vi "LSMcontroller_v57.vi"() -> ()   [LabVIEW 2015] (continued)
                                n403 = Boolean Array To Number(Boolean array=w2608) -> (number=w2607:u32)
                                n404 = case shown="2" w2607 {
                                tunnel: w2604 -> [_ w2650 _ w2657]
                                tunnel: [_ w2649 _ w2655] -> w2603
                                frame 1 {
                                n405 = call "2pparameters.vi"("command"="get") -> ("params out"=w2615:T12)  [unwired: 1 in]
                                n406 = Unbundle By Name(w2615) -> ("wavdet"=w2616:bool, "sAOxy"=w2618:i32, "refwfsize"=w2619:dbl, "srate Img"=w2617:sgl)
                                n407 = call "waveformsDObuffer.vi"("command"="get") -> ("DO wf out"=w2611:digitalwaveform[])  [unwired: 1 in]
                                n408 = case shown="False" w2616 {
                                tunnel: [w2624 w2634] -> w2613
                                tunnel: w2617 -> [w2629 w2645]
                                tunnel: w2618 -> [w2623 w2638]
                                tunnel: w2619 -> [_ w2642]
                                frame False {
                                w2627 = u16 0 items=["unsigned binary", "offset binary", "2's complement"] ("data format (offset binary)")
                                n409 = Initialize Array(sgl 1.0, w2623) -> (w2620:sgl[])
                                n410 = Reciprocal(x=w2629) -> (1/x=w2630:sgl)
                                n411 = Bundle By Name("Y"=w2620, "dt"=w2630) -> (w2625:waveform(sgl))  [unwired: 1 in]
                                n412 = call-poly <vilib>:"Analog to Digital.vi"("data format (offset binary)"=w2627, "compress digital (T)"=TRUE, "full-scale range (pk-pk)"=1.0, "resolution (16 bit)"=1, "analog waveform"=w2625) -> ("digital waveform"=w2624:digitalwaveform)  [unwired: 3 in, 3 out]
                                }
                                frame True {
                                w2637 = u16 0 items=["unsigned binary", "offset binary", "2's complement"] ("data format (offset binary)")
                                n413 = To Double Precision Float(number=w2638) -> (double precision float=w2643:dbl)
                                n414 = Initialize Array(sgl 1.0, w2638) -> (w2631:sgl[])
                                n415 = Divide(x=w2642, y=w2643) -> (x/y=w2640:dbl)
                                n416 = Round Toward +Infinity(x=w2640) -> (ceil(x): smallest int >= x=w2641:dbl)
                                n417 = for {
                                N: w2641 -> [_]
                                tunnel: w2631 -> [w2647]
                                tunnel: [w2647] -> w2644 mode=concatenating
                                }
                                n418 = Reciprocal(x=w2645) -> (1/x=w2646:sgl)
                                n419 = Bundle By Name("Y"=w2644, "dt"=w2646) -> (w2635:waveform(sgl))  [unwired: 1 in]
                                n420 = call-poly <vilib>:"Analog to Digital.vi"("data format (offset binary)"=w2637, "compress digital (T)"=TRUE, "full-scale range (pk-pk)"=1.0, "resolution (16 bit)"=1, "analog waveform"=w2635) -> ("digital waveform"=w2634:digitalwaveform)  [unwired: 3 in, 3 out]
                                }
                                }
                                n421 = Build Array (concatenate)(w2611, w2613) -> (w2609:digitalwaveform[])
                                n422 = call "waveformsDObuffer.vi"("DO wf in"=w2609, "command"="set") -> ()  [unwired: 1 out]
                                }
                                frame 2 {
                                n423 = call "waveformsDObuffer.vi"("command"="get") -> ("DO wf out"=w2652:digitalwaveform[])  [unwired: 1 in]
                                n424 = Delete From Array(array=w2652, length=1, index=w2650) -> (deleted portion=w2649:digitalwaveform[], array with subset deleted=w2648:digitalwaveform[])
                                n425 = call "waveformsDObuffer.vi"("DO wf in"=w2648, "command"="set") -> ()  [unwired: 1 out]
                                }
                                frame 3, Default {
                                }
                                frame 0 {
                                n426 = call "2pparameters.vi"("command"="get") -> ("params out"=w2659:T12)  [unwired: 1 in]
                                n427 = Unbundle By Name(w2659) -> ("autoshutter"=w2658:bool, "wavdet"=w2656:bool)
                                n428 = case shown="True" w2658 {
                                tunnel: w2657 -> [_ w2663]
                                tunnel: w2656 -> [_ w2662]
                                tunnel: [_ w2661] -> w2655
                                frame False {
                                }
                                frame True {
                                n429 = case shown="False" w2662 {
                                tunnel: w2663 -> [w2667 _]
                                tunnel: [w2665 _] -> w2661
                                frame False {
                                w2674 = u16 0 items=["unsigned binary", "offset binary", "2's complement"] ("data format (offset binary)")
                                n430 = call "2pparameters.vi"("command"="get") -> ("params out"=w2681:T12)  [unwired: 1 in]
                                n431 = Unbundle By Name(w2681) -> ("sAOxy"=w2683:i32, "srate Img"=w2682:sgl)
                                n432 = call "waveformsDObuffer.vi"("command"="get") -> ("DO wf out"=w2668:digitalwaveform[])  [unwired: 1 in]
                                n433 = Index Array(array=w2668, index=w2667) -> (element=w2666:digitalwaveform)
                                n434 = Build Array(w2666) -> (w2665:digitalwaveform[])
                                n435 = Initialize Array(sgl 1.0, w2683) -> (w2669:sgl[])
                                n436 = Reciprocal(x=w2682) -> (1/x=w2676:sgl)
                                n437 = Bundle By Name("Y"=w2669, "dt"=w2676) -> (w2672:waveform(sgl))  [unwired: 1 in]
                                n438 = call-poly <vilib>:"Analog to Digital.vi"("data format (offset binary)"=w2674, "compress digital (T)"=TRUE, "full-scale range (pk-pk)"=1.0, "resolution (16 bit)"=1, "analog waveform"=w2672) -> ("digital waveform"=w2679:digitalwaveform)  [unwired: 3 in, 3 out]
                                n439 = Replace Array Subset(array=w2668, new element=w2679, index=w2667) -> (w2664:digitalwaveform[])
                                n440 = call "waveformsDObuffer.vi"("DO wf in"=w2664, "command"="set") -> ()  [unwired: 1 out]
                                }
                                frame True {
                                }
                                }
                                }
                                }
                                }
                                }
                              }
                              frame #8 {
                                n441 = Build Array(w2687, w2686) -> (w2689:bool[])
                                n442 = Boolean Array To Number(Boolean array=w2689) -> (number=w2688:u32)
                                n443 = case shown="0" w2688 {
                                tunnel: w2685 -> [_ w2715 _ w2727]
                                tunnel: [_ w2714 _ w2725] -> w2684
                                frame 1 {
                                w2702 = 0.0 ("DOtab")
                                n444 = call "2pparameters.vi"("command"="get") -> ("params out"=w2700:T12)  [unwired: 1 in]
                                n445 = call "waveformparamsv2.vi"("command"="get") -> ("Params out"=w2710:T16)  [unwired: 4 in, 2 out]
                                n446 = Unbundle By Name(w2710) -> ("DO parameters"=w2708:T19)
                                n447 = Unbundle By Name(w2700) -> ("srate"=w2697:sgl, "sAOxy"=w2699:i32)
                                n448 = To Double Precision Float(number=w2697) -> (double precision float=w2695:dbl)
                                n449 = To Double Precision Float(number=w2697) -> (double precision float=w2696:dbl)
                                n450 = To Double Precision Float(number=w2699) -> (double precision float=w2691:dbl)
                                n451 = Divide(x=w2696, y=w2691) -> (x/y=w2698:dbl)
                                n452 = Index Array(array=w2708, index=0) -> (element=w2707:T20)
                                n453 = Divide(x=1.0 ("Digital DC (%)"), y=w2691) -> (x/y=w2693:dbl)
                                n454 = Multiply(x=100.0, y=w2693) -> (x*y=w2690:dbl)
                                n455 = Bundle By Name(cluster=w2707, "Digital DC (%)"=w2690, "Digital phase"=w2702, "Digital Freq (Hz)"=w2698, "Sampling frequency (Hz)"=w2695, "Digital time offset (s)"=w2702, "padding value"=0.0, "matlab wave file"=path "LT", "DOtab"=0.0) -> (w2705:T20)
                                n456 = Build Array(w2705) -> (w2704:T19)
                                n457 = call "waveformparamsv2.vi"("command"="add DO", "add DO"=w2704) -> ()  [unwired: 3 in, 3 out]
                                }
                                frame 2 {
                                n458 = call "waveformparamsv2.vi"("command"="get") -> ("Params out"=w2717:T16)  [unwired: 4 in, 2 out]
                                n459 = in-place {
                                in-place-border: w2715 -> [w2721]
                                in-place-border: [w2720] -> w2714
                                n460 = in-place-cluster #8(w2717) -> ("DO parameters"=w2723:T19)
                                n461 = Delete From Array(array=w2723, length=1, index=w2721) -> (deleted portion=w2720:T19, array with subset deleted=w2722:T19)
                                n462 = in-place-cluster #8("DO parameters"=w2722) -> (w2716:T16)
                                }
                                n463 = call "waveformparamsv2.vi"("command"="set", "Params in"=w2716) -> ()  [unwired: 3 in, 3 out]
                                }
                                frame 3, Default {
                                }
                                frame 0 {
                                n464 = local read "Measurement"() -> (w2729:T5)
                                n465 = To Unsigned Long Integer(number=w2729) -> (unsigned 32bit integer=w2728:u32)
                                n466 = case shown="5..7" w2728 {
                                tunnel: w2727 -> [_ w2731]
                                tunnel: [_ w2730] -> w2726
                                frame 0..4, Default {
                                }
                                frame 5..7 {
                                n467 = stacked-sequence {
                                tunnel: w2731 -> [w2733 w2742]
                                tunnel: [w2732 _] -> w2730
                                frame #0 {
                                n468 = call "waveformparamsv2.vi"("command"="get") -> ("Params out"=w2735:T16)  [unwired: 4 in, 2 out]
                                n469 = Unbundle By Name(w2735) -> ("DO parameters"=w2736:T19)
                                n470 = Index Array(array=w2736, index=w2733) -> (element=w2732:T20)
                                }
                                frame #1 {
                                w2750 = 0.0 ("padding value")
                                n471 = call "2pparameters.vi"("command"="get") -> ("params out"=w2748:T12)  [unwired: 1 in]
                                n472 = Unbundle By Name(w2748) -> ("srate"=w2746:sgl, "sAOxy"=w2747:i32)
                                n473 = To Double Precision Float(number=w2746) -> (double precision float=w2744:dbl)
                                n474 = To Double Precision Float(number=w2746) -> (double precision float=w2745:dbl)
                                n475 = To Double Precision Float(number=w2747) -> (double precision float=w2740:dbl)
                                n476 = Divide(x=1.0 ("Digital DC (%)"), y=w2740) -> (x/y=w2739:dbl)
                                n477 = Multiply(x=100.0, y=w2739) -> (x*y=w2738:dbl)
                                n478 = Divide(x=w2745, y=w2740) -> (x/y=w2743:dbl)
                                n479 = call "replace DO wf param.vi"("Digital Freq (Hz)"=w2743, "Digital DC (%)"=w2738, "Digital phase"=w2750, "Sampling frequency (Hz)"=w2744, "Digital time offset (s)"=w2750, "index of DO wave"=w2742, "padding value"=w2750, "matlab wave file"=path "LT" ("matlab wave number")) -> ()  [unwired: 3 in]
                                }
                                }
                                }
                                }
                                n480 = Build Array(w2726) -> (w2725:T19)
                                }
                                }
                              }
                              frame #9 {
                                n481 = Build Array(w2755, w2754) -> (w2757:bool[])
                                n482 = Boolean Array To Number(Boolean array=w2757) -> (number=w2756:u32)
                                n483 = case shown="2" w2756 {
                                tunnel: w2753 -> [_ w2809 _ w2813]
                                tunnel: [_ w2804 _ w2810] -> w2752
                                frame 1 {
                                n484 = call "2pparameters.vi"("command"="get") -> ("params out"=w2764:T12)  [unwired: 1 in]
                                n485 = Unbundle By Name(w2764) -> ("wavdet"=w2765:bool, "sAOxy"=w2767:i32, "refwfsize"=w2768:dbl, "srate Img"=w2766:sgl)
                                n486 = call "waveformsDObuffer.vi"("command"="get") -> ("DO wf out"=w2760:digitalwaveform[])  [unwired: 1 in]
                                n487 = case shown="True" w2765 {
                                tunnel: [w2772 w2785] -> w2762
                                tunnel: w2766 -> [w2781 w2800]
                                tunnel: w2767 -> [w2771 w2791]
                                tunnel: w2768 -> [_ w2797]
                                frame False {
                                w2775 = u16 0 items=["unsigned binary", "offset binary", "2's complement"] ("data format (offset binary)")
                                n488 = Initialize Array(sgl 0.0, w2771) -> (w2778:sgl[])
                                n489 = Replace Array Subset(array=w2778, new element=sgl 1.0, index=0) -> (w2776:sgl[])
                                n490 = Reciprocal(x=w2781) -> (1/x=w2782:sgl)
                                n491 = Bundle By Name("Y"=w2776, "dt"=w2782) -> (w2773:waveform(sgl))  [unwired: 1 in]
                                n492 = call-poly <vilib>:"Analog to Digital.vi"("data format (offset binary)"=w2775, "compress digital (T)"=TRUE, "full-scale range (pk-pk)"=1.0, "resolution (16 bit)"=1, "analog waveform"=w2773) -> ("digital waveform"=w2772:digitalwaveform)  [unwired: 3 in, 3 out]
                                }
                                frame True {
                                w2788 = u16 0 items=["unsigned binary", "offset binary", "2's complement"] ("data format (offset binary)")
                                n493 = To Double Precision Float(number=w2791) -> (double precision float=w2798:dbl)
                                n494 = Initialize Array(sgl 0.0, w2791) -> (w2793:sgl[])
                                n495 = Divide(x=w2797, y=w2798) -> (x/y=w2795:dbl)
                                n496 = Round Toward +Infinity(x=w2795) -> (ceil(x): smallest int >= x=w2796:dbl)
                                n497 = Replace Array Subset(array=w2793, new element=sgl 1.0, index=0) -> (w2790:sgl[])
                                n498 = for {
                                N: w2796 -> [_]
                                tunnel: w2790 -> [w2802]
                                tunnel: [w2802] -> w2799 mode=concatenating
                                }
                                n499 = Reciprocal(x=w2800) -> (1/x=w2801:sgl)
                                n500 = Bundle By Name("Y"=w2799, "dt"=w2801) -> (w2786:waveform(sgl))  [unwired: 1 in]
                                n501 = call-poly <vilib>:"Analog to Digital.vi"("data format (offset binary)"=w2788, "compress digital (T)"=TRUE, "full-scale range (pk-pk)"=1.0, "resolution (16 bit)"=1, "analog waveform"=w2786) -> ("digital waveform"=w2785:digitalwaveform)  [unwired: 3 in, 3 out]
                                }
                                }
                                n502 = Build Array (concatenate)(w2760, w2762) -> (w2758:digitalwaveform[])
                                n503 = call "waveformsDObuffer.vi"("DO wf in"=w2758, "command"="set") -> ()  [unwired: 1 out]
                                }
                                frame 2 {
                                n504 = call "waveformsDObuffer.vi"("command"="get") -> ("DO wf out"=w2806:digitalwaveform[])  [unwired: 1 in]
                                n505 = Delete From Array(array=w2806, length=1, index=w2809) -> (deleted portion=w2804:digitalwaveform[], array with subset deleted=w2803:digitalwaveform[])
                                n506 = call "waveformsDObuffer.vi"("DO wf in"=w2803, "command"="set") -> ()  [unwired: 1 out]
                                }
                                frame 3, Default {
                                }
                                frame 0 {
                                n507 = local read "Measurement"() -> (w2812:T5)
                                n508 = To Unsigned Long Integer(number=w2812) -> (unsigned 32bit integer=w2811:u32)
                                n509 = case shown="5..7" w2811 {
                                tunnel: w2813 -> [_ w2816]
                                tunnel: [_ w2815] -> w2810
                                frame 0..4, Default {
                                }
                                frame 5..7 {
                                n510 = call "2pparameters.vi"("command"="get") -> ("params out"=w2823:T12)  [unwired: 1 in]
                                n511 = Unbundle By Name(w2823) -> ("wavdet"=w2824:bool, "sAOxy"=w2826:i32, "refwfsize"=w2827:dbl, "srate Img"=w2825:sgl)
                                n512 = call "waveformsDObuffer.vi"("command"="get") -> ("DO wf out"=w2817:digitalwaveform[])  [unwired: 1 in]
                                n513 = Index Array(array=w2817, index=w2816) -> (element=w2818:digitalwaveform)
                                n514 = case shown="True" w2824 {
                                tunnel: [w2831 w2844] -> w2821
                                tunnel: w2825 -> [w2840 w2859]
                                tunnel: w2826 -> [w2830 w2850]
                                tunnel: w2827 -> [_ w2856]
                                frame False {
                                w2834 = u16 0 items=["unsigned binary", "offset binary", "2's complement"] ("data format (offset binary)")
                                n515 = Initialize Array(sgl 0.0, w2830) -> (w2837:sgl[])
                                n516 = Replace Array Subset(array=w2837, new element=sgl 1.0, index=0) -> (w2835:sgl[])
                                n517 = Reciprocal(x=w2840) -> (1/x=w2841:sgl)
                                n518 = Bundle By Name("Y"=w2835, "dt"=w2841) -> (w2832:waveform(sgl))  [unwired: 1 in]
                                n519 = call-poly <vilib>:"Analog to Digital.vi"("data format (offset binary)"=w2834, "compress digital (T)"=TRUE, "full-scale range (pk-pk)"=1.0, "resolution (16 bit)"=1, "analog waveform"=w2832) -> ("digital waveform"=w2831:digitalwaveform)  [unwired: 3 in, 3 out]
                                }
                                frame True {
                                w2847 = u16 0 items=["unsigned binary", "offset binary", "2's complement"] ("data format (offset binary)")
                                n520 = To Double Precision Float(number=w2850) -> (double precision float=w2857:dbl)
                                n521 = Initialize Array(sgl 0.0, w2850) -> (w2852:sgl[])
                                n522 = Divide(x=w2856, y=w2857) -> (x/y=w2854:dbl)
                                n523 = Round Toward +Infinity(x=w2854) -> (ceil(x): smallest int >= x=w2855:dbl)
                                n524 = Replace Array Subset(array=w2852, new element=sgl 1.0, index=0) -> (w2849:sgl[])
                                n525 = for {
                                N: w2855 -> [_]
                                tunnel: w2849 -> [w2861]
                                tunnel: [w2861] -> w2858 mode=concatenating
                                }
                                n526 = Reciprocal(x=w2859) -> (1/x=w2860:sgl)
                                n527 = Bundle By Name("Y"=w2858, "dt"=w2860) -> (w2845:waveform(sgl))  [unwired: 1 in]
                                n528 = call-poly <vilib>:"Analog to Digital.vi"("data format (offset binary)"=w2847, "compress digital (T)"=TRUE, "full-scale range (pk-pk)"=1.0, "resolution (16 bit)"=1, "analog waveform"=w2845) -> ("digital waveform"=w2844:digitalwaveform)  [unwired: 3 in, 3 out]
                                }
                                }
                                n529 = Build Array(w2818) -> (w2815:digitalwaveform[])
                                n530 = Replace Array Subset(array=w2817, new element=w2821, index=w2816) -> (w2814:digitalwaveform[])
                                n531 = call "waveformsDObuffer.vi"("DO wf in"=w2814, "command"="set") -> ()  [unwired: 1 out]
                                }
                                }
                                }
                                }
                              }
                              frame #10 {
                                n532 = local read "Meastab"() -> (w2876:enum32{"X-Y Image", "Linescan", "Timetrace"})
                                n533 = property on="refwf" class="Ring (strict)"() -> ("RingText.Text"=w2873:string)  [unwired: 2 in, 2 out]
                                n534 = case shown="\"Timetrace\"" w2876 {
                                tunnel: [w2878 w2879] -> w2877
                                frame "X-Y Image", Default {
                                n535 = local read "Sampling rate"() -> (w2878:dbl)
                                }
                                frame "Timetrace" {
                                n536 = local read "srateAODOtt"() -> (w2879:dbl)
                                }
                                }
                                n537 = call "waveformsAObuffer.vi"("command"="get") -> ("AO wf out"=w2864:waveform(dbl)[])  [unwired: 1 in]
                                n538 = local read "wavdet"() -> (w2874:bool)
                                n539 = call "waveformsDObuffer.vi"("command"="get") -> ("DO wf out"=w2868:digitalwaveform[])  [unwired: 1 in]
                                n540 = call "correctwaveformsizetemp.vi"("new sampling frequency (Hz)"=w2877, "start"=TRUE, "reference waveforms to"=w2873, "Analog waveforms in"=w2864, "stop"=FALSE, "Digital waveforms in"=w2868) -> ("analog wf out"=w2870:waveform(dbl)[], "Digital wf out"=w2872:digitalwaveform[], "measpoints"=w2875:i32)
                                n541 = call "GetNumCamFramesv2.vi"("Digital Waveform Graph"=w2872) -> ("Numeric"=w2871:i32)  [unwired: 10 in]
                                n542 = call "waveformsDObuffer.vi"("DO wf in"=w2872, "command"="set") -> ()  [unwired: 1 out]
                                n543 = call "waveformsAObuffer.vi"("AO wf in"=w2870, "command"="set") -> ()  [unwired: 1 out]
                                n544 = local write "Total Camera Frames"(w2871) -> ()
                                n545 = case shown="True" w2874 {
                                tunnel: w2875 -> [_ w2880]
                                frame False {
                                }
                                frame True {
                                n546 = local write "# of frames"(w2880) -> ()
                                }
                                }
                              }
                            }
                          }
                          frame #6 {
                            # "Disabled for conversion to 64 bit"
                            n547 = disable-structure shown="Disabled" {
                              frame Disabled {
                                n548 = local read "Measurement"() -> (w2885:T5)
                                n549 = case shown="\"Lifetime (scan)\"" w2885 {
                                frame "X-Y-t movie", Default {
                                }
                                frame "Lifetime (scan)" {
                                # "total acquisition time"
                                n550 = call "2pparameters.vi"("command"="get") -> ("params out"=w2891:T12)  [unwired: 1 in]
                                n551 = Unbundle By Name(w2891) -> ("measpoints"=w2912:i32, "avpp"=w2913:i32, "sAOxy"=w2892:i32, "srate Img"=w2914:sgl)
                                n552 = Multiply(x=w2912, y=w2913) -> (x*y=w2910:i32)
                                n553 = To Double Precision Float(number=w2892) -> (double precision float=w2897:dbl)
                                n554 = Divide(x=w2897, y=w2914) -> (x/y=w2899:dbl)
                                n555 = To Double Precision Float(number=w2910) -> (double precision float=w2895:dbl)
                                n556 = local read "min phot"() -> (w2906:u32)
                                n557 = local read "expected c/s"() -> (w2907:dbl)
                                n558 = Multiply(x=w2895, y=w2899) -> (x*y=w2893:dbl)
                                n559 = Multiply(x=w2893, y=1000.0) -> (x*y=w2898:dbl)
                                n560 = local read "Ch1 ZeroX"() -> (w2904:i32)
                                n561 = local read "truncate"() -> (w2905:u32)
                                n562 = To Long Integer(number=w2898) -> (32bit integer=w2908:i32)
                                n563 = To Long Integer(number=w2907) -> (32bit integer=w2909:i32)
                                n564 = local read "Number of Bins"() -> (w2900:u32)
                                n565 = local read "Ch1 Level"() -> (w2902:i32)
                                n566 = local read "Ch0 ZeroX"() -> (w2903:i32)
                                n567 = local write "Acquisition time"(w2908) -> ()
                                n568 = local read "Ch0 Level"() -> (w2901:i32)
                                n569 = call "lifetimeparameters.vi"("command"="get") -> ("Params out"=w2889:T21)  [unwired: 1 in]
                                n570 = Add(x=10, y=w2908) -> (x+y=w2896:i32)
                                n571 = Bundle By Name(cluster=w2889, "acq time"=w2896, "acq rate"=w2909, "# bins"=w2900, "Ch0 Level"=w2901, "Ch1 Level"=w2902, "Ch0 ZeroX"=w2903, "Ch1 ZeroX"=w2904, "min photons"=w2906, "truncate"=w2905) -> (w2888:T21)
                                n572 = local write "Acquisition rate"(w2909) -> ()
                                n573 = call "lifetimeparameters.vi"("Params in"=w2888, "command"="set") -> ()  [unwired: 1 out]
                                }
                                }
                                n574 = local read "min phot"() -> (w2883:u32)
                                n575 = Decrement(x=w2883) -> (x-1=w2884:u32)
                                n576 = To Double Precision Float(number=w2884) -> (double precision float=w2882:dbl)
                                n577 = property on="img_CH1" class="IntGraph (strict)"("ZScale.Minimum"=w2882) -> ()  [unwired: 2 in, 2 out]
                              }
                              frame Enabled {
                              }
                            }
                            n578 = local write "64bit disabled"(TRUE ("64bit disabled")) -> ()
                          }
                          frame #7 {
                            n579 = local read "Sampling rate"() -> (w2916:dbl)
                            n580 = call "calcdaqtime.vi"("sampling rate"=w2916) -> ("Calc. time per frame (ms)"=w2915:dbl)
                            n581 = local write "Calc. time per frame (ms)"(w2915) -> ()
                          }
                          frame #8 {
                            n582 = call "2pparameters.vi"("command"="get") -> ("params out"=w2927:T12)  [unwired: 1 in]
                            n583 = local read "Measurement"() -> (w2918:T5)
                            n584 = Unbundle By Name(w2927) -> ("bufferAI"=w2925:i32, "srate"=w2926:sgl)
                            n585 = To Double Precision Float(number=w2925) -> (double precision float=w2919:dbl)
                            n586 = To Double Precision Float(number=w2926) -> (double precision float=w2929:dbl)
                            n587 = case shown="\"X-Y-t movie\", Default" w2918 {
                              tunnel: [w2934 w2938] -> w2917
                              frame "X-Y-t movie", Default {
                                n588 = local read "wavdet"() -> (w2935:bool)
                                n589 = case shown="False" w2935 {
                                tunnel: [w2936 w2937] -> w2934
                                frame False {
                                w2936 = 10123 items=["Finite Samples"=10178, "Continuous Samples"=10123, "Hardware Timed Single Point"=12522] ("sample mode")
                                }
                                frame True {
                                w2937 = 10123 items=["Finite Samples"=10178, "Continuous Samples"=10123, "Hardware Timed Single Point"=12522] ("sample mode")
                                }
                                }
                              }
                              frame "X-Y-Z stack" {
                                w2938 = 10178 items=["Finite Samples"=10178, "Continuous Samples"=10123, "Hardware Timed Single Point"=12522] ("sample mode")
                              }
                            }
                            n590 = Divide(x=w2919, y=w2929) -> (x/y=w2933:dbl)
                            n591 = Multiply(x=w2933, y=2.0) -> (x*y=w2930:dbl)
                            n592 = Max & Min(x=w2930, y=10.0) -> (max(x,y)=w2920:dbl)  [unwired: 1 out]
                            n593 = call "2pparameters.vi"("command"="get") -> ("params out"=w2924:T12)  [unwired: 1 in]
                            n594 = Bundle By Name(cluster=w2924, "timeout"=w2920, "sample mode"=w2917) -> (w2921:T12)
                            n595 = call "2pparameters.vi"("Params in"=w2921, "command"="set") -> ()  [unwired: 1 out]
                          }
                          frame #9 {
                            n596 = local read "# of frames"() -> (w2939:i32)
                            n597 = call "timestamps.vi"("# of frames"=w2939, "command"="init") -> ()  [unwired: 2 in, 1 out]
                          }
                        }
                      }
                      frame #2 {
                        # "Disabled for conversion to 64 bit"
                        n598 = call "prepAO_img.vi"() -> ("Terminal Name with Device Prefix"=w2942:tag)
                        n599 = call "prepAI_img.vi"("triggersource"=w2942) -> ()  [unwired: 2 in]
                        n600 = call "prepCI_img.vi"("ArmStart.DigEdge.Src"=w2942) -> ()  [unwired: 1 in]
                        n601 = call "prepDO_img.vi"() -> ()  [unwired: 2 in]
                        n602 = disable-structure shown="Disabled" {
                          frame Disabled {
                            n603 = local read "Measurement"() -> (w2943:T5)
                            n604 = case shown="\"Lifetime (scan)\"" w2943 {
                              frame "X-Y-t movie", Default {
                              }
                              frame "Lifetime (scan)" {
                                n605 = stacked-sequence {
                                frame #0 {
                                n606 = call "PH-temp.vi"("String"="clear" ("command")) -> ()  [unwired: 2 in, 2 out]
                                n607 = call "PH-temp-raw.vi"("command"="empty") -> ()  [unwired: 1 in, 1 out]
                                }
                                frame #1 {
                                n608 = call "calib.vi"() -> ()  [unwired: 1 in]
                                }
                                frame #2 {
                                n609 = call "setup.vi"() -> ()  [unwired: 1 in]
                                }
                                }
                              }
                            }
                          }
                          frame Enabled {
                          }
                        }
                        n610 = local write "64bit disabled"(TRUE ("64bit disabled")) -> ()
                      }
                      frame #3 {
                        n611 = local read "save\ndata"() -> (w2946:bool)
                        n612 = case shown="True" w2946 {
                          tunnel: w2947 -> [_ w2951]
                          frame False {
                          }
                          frame True {
                            n613 = local read "filename prefix"() -> (w2949:string)
                            n614 = local read "data dir"() -> (w2950:path)
                            n615 = call "preparetiffs.vi"("filename prefix"=w2949, "data dir"=w2950, "timestamp"=w2951) -> ("full-filename"=w2948:string)  [unwired: 1 in]
                            n616 = local write "full-filename"(w2948) -> ()
                          }
                        }
                        n617 = call "preptempbuffers.vi"() -> ()  [unwired: 12 in]
                      }
                      frame #4 {
                        # "Disabled Thorlabs Zstage;\nneeds to be replaced by PI code"
                        n618 = disable-structure shown="Disabled" {
                          frame Disabled {
                            n619 = local read "Measurement"() -> (w2953:T5)
                            n620 = case shown="\"X-Y-Z stack\"" w2953 {
                              frame "X-Y-t movie", Default {
                              }
                              frame "X-Y-Z stack" {
                                n621 = local read "Z-Start (um)"() -> (w2964:dbl)
                                n622 = local read "Z-end (um)"() -> (w2963:dbl)
                                n623 = local read "# of frames"() -> (w2965:i32)
                                n624 = call "2pparameters.vi"("command"="get") -> ("params out"=w2956:T12)  [unwired: 1 in]
                                n625 = Unbundle By Name(w2956) -> ("motorref"=w2955:refnum<k7>)
                                n626 = call "calcZslice.vi"("current slice"=0, "# of Slices"=w2965, "Z-Start (um)"=w2964, "Z-end (um)"=w2963) -> ("zpos (mm)"=w2958:sgl)
                                n627 = call "MoveZ.vi"("RetPos"=TRUE, "Wait"=TRUE, "GoTo (mm)"=w2958, "MG17Motor"=w2955) -> ("EndPosition (um)"=w2962:sgl)  [unwired: 1 out]
                                n628 = Multiply(x=w2958, y=sgl 1000.0) -> (x*y=w2959:sgl)
                                n629 = local write "Actual Z position"(w2962) -> ()
                                n630 = local write "Cal. Z"(w2959) -> ()
                              }
                            }
                          }
                          frame Enabled {
                          }
                        }
                        n631 = local write "Thorlabs Zstage disabled"(TRUE ("64bit disabled")) -> ()
                      }
                      frame #5 {
                        n632 = flat-sequence {
                          frame #0 {
                            n633 = call "2pparameters.vi"("command"="get") -> ("params out"=w2968:T12)  [unwired: 1 in]
                            n634 = Unbundle By Name(w2968) -> ("autoshutter"=w2969:bool)
                            n635 = case shown="True" w2969 {
                              frame False {
                              }
                              frame True {
                                n636 = call "shuttercontrol.vi"("command"="open") -> ()  [unwired: 1 in, 1 out]
                              }
                            }
                          }
                          frame #1 {
                            n637 = call "2pparameters.vi"("command"="get") -> ("params out"=w2973:T12)  [unwired: 1 in]
                            n638 = Tick Count (ms)() -> (millisecond timer value=w2972:u32)
                            n639 = Bundle By Name(cluster=w2973, "starttick"=w2972) -> (w2971:T12)
                            n640 = call "2pparameters.vi"("Params in"=w2971, "command"="set") -> ()  [unwired: 1 out]
                          }
                        }
                      }
                      frame #6 {
                        n641 = local read "Measurement"() -> (w2976:T5)
                        n642 = case shown="\"Lifetime (scan)\"" w2976 {
                          frame "X-Y-t movie" {
                            n643 = flat-sequence {
                              frame #0 {
                                n644 = call "runAI_img.vi"() -> ()  [unwired: 12 in]
                                n645 = call "runCI.vi"() -> ()  [unwired: 12 in]
                                n646 = call "runDO_img.vi"() -> ()  [unwired: 12 in]
                              }
                              frame #1 {
                                n647 = call "runAO_img.vi"() -> ()  [unwired: 12 in]
                              }
                            }
                          }
                          frame "Lifetime (scan)" {
                            # "Disabled for conversion to 64 bit"
                            n648 = disable-structure shown="Disabled" {
                              frame Disabled {
                                n649 = flat-sequence {
                                frame #0 {
                                n650 = call "runLT_img.vi"() -> ()  [unwired: 1 in]
                                n651 = call "runDO_img.vi"() -> ()  [unwired: 12 in]
                                }
                                frame #1 {
                                n652 = call "runAI_img.vi"() -> ()  [unwired: 12 in]
                                n653 = call "runCI.vi"() -> ()  [unwired: 12 in]
                                }
                                frame #2 {
                                n654 = call "runAO_img.vi"() -> ()  [unwired: 12 in]
                                }
                                }
                              }
                              frame Enabled {
                              }
                            }
                            n655 = local write "64bit disabled"(TRUE ("64bit disabled")) -> ()
                          }
                          frame "X-Y-Z stack", Default {
                          }
                        }
                      }
                      frame #7 {
                        # "Disabled for conversion to 64 bit"
                        n656 = while {
                          i -> [w3005]
                          stop <- w3002 stop-if-true
                          n657 = local read "Exit"() -> (w3010:bool)
                          n658 = local read "Stop"() -> (w3001:bool)
                          n659 = Or(x=w3001, y=w3010) -> (x .or. y?=w3006:bool)
                          n660 = case shown="False" w3006 {
                            tunnel: w3005 -> [w3011 _]
                            frame False {
                              n661 = stacked-sequence {
                                seq-local: [w3013 _ _ _ _ _ _] -> [_ _ _ _ _ _ w3138]
                                seq-local: [w3012 _ _ _ _ _ _] -> [_ _ _ _ _ _ w3137]
                                tunnel: w3011 -> [_ w3018 _ _ _ _ _]
                                frame #0 {
                                n662 = local read "Live"() -> (w3014:bool)
                                n663 = case shown="True" w3014 {
                                tunnel: [_ w3016] -> w3013
                                tunnel: [_ w3015] -> w3012
                                frame False {
                                }
                                frame True {
                                n664 = local read "Laserpower \n(%)"() -> (w3015:dbl)
                                n665 = local read "lpow"() -> (w3016:dbl)
                                }
                                }
                                n666 = call "preptempbuffers.vi"() -> ()  [unwired: 12 in]
                                }
                                frame #1 {
                                # "Disabled Thorlabs Zstage;\nneeds to be replaced by PI code"
                                n667 = disable-structure shown="Disabled" {
                                disable-tunnel: w3018 -> [w3019 _]
                                frame Disabled {
                                # "Move in Z if necessary"
                                n668 = local read "Measurement"() -> (w3020:T5)
                                n669 = case shown="\"X-Y-Z stack\"" w3020 {
                                tunnel: w3019 -> [_ w3024]
                                frame "X-Y-t movie", Default {
                                }
                                frame "X-Y-Z stack" {
                                n670 = local read "Z-Start (um)"() -> (w3031:dbl)
                                n671 = local read "Z-end (um)"() -> (w3030:dbl)
                                n672 = local read "# of frames"() -> (w3032:i32)
                                n673 = call "2pparameters.vi"("command"="get") -> ("params out"=w3022:T12)  [unwired: 1 in]
                                n674 = Unbundle By Name(w3022) -> ("motorref"=w3021:refnum<k7>)
                                n675 = call "calcZslice.vi"("current slice"=w3024, "# of Slices"=w3032, "Z-Start (um)"=w3031, "Z-end (um)"=w3030) -> ("zpos (mm)"=w3025:sgl)
                                n676 = call "MoveZ.vi"("RetPos"=TRUE, "Wait"=TRUE, "GoTo (mm)"=w3025, "MG17Motor"=w3021) -> ("EndPosition (um)"=w3029:sgl)  [unwired: 1 out]
                                n677 = Multiply(x=w3025, y=sgl 1000.0) -> (x*y=w3026:sgl)
                                n678 = local write "Actual Z position"(w3029) -> ()
                                n679 = local write "Cal. Z"(w3026) -> ()
                                }
                                }
                                }
                                frame Enabled {
                                }
                                }
                                n680 = local write "Thorlabs Zstage disabled"(TRUE ("64bit disabled")) -> ()
                                }
                                frame #2 {
                                # "main loop"
                                n681 = for {
                                N: "avpp" -> [_]
                                i -> [w3039]
                                n682 = local read "Stop"() -> (w3037:bool)
                                n683 = local read "Exit"() -> (w3036:bool)
                                n684 = Increment(x=w3039) -> (x+1=w3038:i32)
                                n685 = Or(x=w3037, y=w3036) -> (x .or. y?=w3035:bool)
                                n686 = case shown="False" w3035 {
                                tunnel: w3038 -> [w3040 _]
                                frame False {
                                n687 = stacked-sequence {
                                seq-local: [w3041 _ _ _ _ _ _] -> [_ _ _ w3054 w3066 w3074 _]
                                tunnel: w3040 -> [w3042 _ _ _ _ _ _]
                                frame #0 {
                                n688 = local read "Live"() -> (w3041:bool)
                                n689 = case shown="True" w3041 {
                                tunnel: w3042 -> [_ w3045]
                                frame False {
                                }
                                frame True {
                                # "collect timetag for current image\nplus curent average"
                                n690 = To Single Precision Float(number=w3045) -> (single precision float=w3043:sgl)
                                n691 = Tick Count (ms)() -> (millisecond timer value=w3044:u32)
                                n692 = local write "Tick for Frame"(w3044) -> ()
                                n693 = local write "Current Average"(w3043) -> ()
                                }
                                }
                                }
                                frame #1 {
                                n694 = local read "Measurement"() -> (w3046:T5)
                                n695 = case shown="\"X-Y-Z stack\"" w3046 {
                                frame "X-Y-t movie", Default {
                                }
                                frame "X-Y-Z stack" {
                                n696 = stacked-sequence {
                                frame #0 {
                                n697 = disable-structure shown="Disabled" {
                                frame Disabled {
                                n698 = call "2pparameters.vi"("command"="get") -> ("params out"=w3048:T12)  [unwired: 1 in]
                                n699 = Unbundle By Name(w3048) -> ("autoshutter"=w3049:bool)
                                n700 = case shown="True" w3049 {
                                frame False {
                                }
                                frame True {
                                n701 = call "shuttercontrol.vi"("command"="open") -> ()  [unwired: 1 in, 1 out]
                                }
                                }
                                }
                                frame Enabled {
                                }
                                }
                                }
                                frame #1 {
                                n702 = call "runAI_img.vi"() -> ()  [unwired: 12 in]
                                n703 = call "runCI.vi"() -> ()  [unwired: 12 in]
                                n704 = call "runDO_img.vi"() -> ()  [unwired: 12 in]
                                }
                                frame #2 {
                                n705 = call "runAO_img.vi"() -> ()  [unwired: 12 in]
                                }
                                }
                                }
                                }
                                }
                                frame #2 {
                                n706 = call "collectCI_img.vi"() -> ("Avg cts/s"=w3053:dbl, "recorded samples"=w3052:i32)  [unwired: 1 out]
                                n707 = call "collectAI_img.vi"() -> ("wrap"=w3051:i32)  [unwired: 3 in]
                                n708 = local write "scol"(w3052) -> ()
                                n709 = local write "wrap"(w3051) -> ()
                                n710 = local write "Avg Counts/s"(w3053) -> ()
                                }
                                frame #3 {
                                n711 = case shown="True" w3054 {
                                frame False {
                                }
                                frame True {
                                n712 = local read "Measurement"() -> (w3055:T5)
                                n713 = case shown="\"X-Y-t movie\", Default" w3055 {
                                frame "X-Y-t movie", Default {
                                n714 = local read "ROI Type"() -> (w3056:u16)
                                n715 = case shown="0" w3056 {
                                frame 0 {
                                # "display chosen channels"
                                n716 = local read "Current Average"() -> (w3065:sgl)
                                n717 = local read "image1list"() -> (w3061:u16)
                                n718 = local read "image2list"() -> (w3064:u16)
                                n719 = To Unsigned Word Integer(number=w3064) -> (unsigned 16bit integer=w3059:u16)
                                n720 = To Unsigned Word Integer(number=w3061) -> (unsigned 16bit integer=w3060:u16)
                                n721 = call "dattoimage.vi"("image2list"=w3059, "Current Average"=w3065, "image1list"=w3060) -> ("image 2 array out"=w3063:sgl[][], "image 1 array out"=w3062:sgl[][])
                                n722 = Transpose 2D Array(2D array=w3062) -> (transposed array=w3058:sgl[][])
                                n723 = Transpose 2D Array(2D array=w3063) -> (transposed array=w3057:sgl[][])
                                n724 = local write "img_CH1"(w3058) -> ()
                                n725 = local write "img_CH2"(w3057) -> ()
                                }
                                frame 1, Default {
                                }
                                }
                                }
                                frame "Lifetime (scan)" {
                                }
                                }
                                }
                                }
                                }
                                frame #4 {
                                n726 = case shown="True" w3066 {
                                frame False {
                                }
                                frame True {
                                # "set colormaps"
                                n727 = call "misc-global.vi"("command"="get") -> ("misc out"=w3070:cluster{"Colormaps":u32[][]})  [unwired: 1 in]
                                n728 = Unbundle By Name(w3070) -> ("Colormaps"=w3069:u32[][])
                                n729 = control-ref of="img_CH1"() -> (w3073:refnum<vi>)
                                n730 = control-ref of="img_CH2"() -> (w3072:refnum<vi>)
                                n731 = Index Array(array=w3069, index (row)="Colormap") -> (element=w3068:u32[])  [unwired: 1 in]
                                n732 = property class="IntGraph (strict)"(reference=w3073, "Color Table"=w3068) -> ()  [unwired: 1 in, 2 out]
                                n733 = property class="IntGraph (strict)"(reference=w3072, "Color Table"=w3068) -> ()  [unwired: 1 in, 2 out]
                                }
                                }
                                }
                                frame #5 {
                                n734 = case shown="True" w3074 {
                                frame False {
                                }
                                frame True {
                                # "crude estimate of time per frame\n(resolution is 1 ms), not so much for\nplotting purposes, more for debugging\ncollection and processing data"
                                n735 = local read "ypixels ref"() -> (w3079:i32)
                                n736 = local read "Tick for Frame"() -> (w3080:u32)
                                n737 = Tick Count (ms)() -> (millisecond timer value=w3081:u32)
                                n738 = To Double Precision Float(number=w3079) -> (double precision float=w3078:dbl)
                                n739 = Subtract(x=w3081, y=w3080) -> (x-y=w3076:u32)
                                n740 = To Double Precision Float(number=w3076) -> (double precision float=w3077:dbl)
                                n741 = local write "Meas. time per frame (ms)"(w3076) -> ()
                                n742 = Divide(x=w3077, y=w3078) -> (x/y=w3075:dbl)
                                n743 = local write "time per line (ms)"(w3075) -> ()
                                }
                                }
                                }
                                frame #6 {
                                n744 = local read "Measurement"() -> (w3082:T5)
                                n745 = case shown="\"X-Y-Z stack\"" w3082 {
                                frame "X-Y-t movie", Default {
                                }
                                frame "X-Y-Z stack" {
                                n746 = call "2pparameters.vi"("command"="get") -> ("params out"=w3084:T12)  [unwired: 1 in]
                                n747 = Unbundle By Name(w3084) -> ("autoshutter"=w3085:bool)
                                n748 = call "stopCI_img.vi"() -> ()  [unwired: 12 in]
                                n749 = call "stopAI_img.vi"() -> ()  [unwired: 12 in]
                                n750 = case shown="True" w3085 {
                                frame False {
                                }
                                frame True {
                                n751 = call "shuttercontrol.vi"("command"="close") -> ()  [unwired: 1 in, 1 out]
                                }
                                }
                                n752 = Wait (ms)(milliseconds to wait=u32 100) -> ()  [unwired: 1 out]
                                n753 = call "stopAO_img.vi"() -> ()  [unwired: 12 in]
                                n754 = call "stopDO_img.vi"() -> ()  [unwired: 12 in]
                                }
                                }
                                }
                                }
                                }
                                frame True {
                                }
                                }
                                }
                                }
                                frame #3 {
                                n755 = local read "Measurement"() -> (w3088:T5)
                                n756 = case shown="\"Lifetime (scan)\"" w3088 {
                                frame "X-Y-t movie", Default {
                                }
                                frame "Lifetime (scan)" {
                                w3091 = u16 2 items=["Stream to disk", "Post process", "real time process"] ("Ring")
                                n757 = local read "T3R Data processing"() -> (w3092:u16)
                                n758 = Equal?(x=w3092, y=w3091) -> (x = y?=w3090:bool)
                                n759 = case shown="True" w3090 {
                                frame False {
                                }
                                frame True {
                                n760 = disable-structure shown="Disabled" {
                                frame Disabled {
                                n761 = local read "lineshift"() -> (w3095:i32)
                                n762 = call "wrapcutlifetime.vi"("lineshift"=w3095) -> ("pt3img"=w3097:u16[][], "lifetimes"=w3096:sgl[][], "okay"=w3093:bool, "# of frames"=w3094:i32)
                                n763 = case shown="True" w3093 {
                                tunnel: w3097 -> [_ w3107]
                                tunnel: w3096 -> [_ w3105]
                                tunnel: w3094 -> [_ w3101]
                                frame False {
                                }
                                frame True {
                                # "lifetime"
                                # "intensity"
                                n764 = Transpose 2D Array(2D array=w3107) -> (transposed array=w3099:u16[][])
                                n765 = Transpose 2D Array(2D array=w3105) -> (transposed array=w3106:sgl[][])
                                n766 = local write "frames recorded"(w3101) -> ()
                                n767 = local read "counts"() -> (w3100:i32)
                                n768 = Array Max & Min(array=w3099) -> (max value=w3104:u16)  [unwired: 3 out]
                                n769 = To Single Precision Float(number=w3099) -> (single precision float=w3098:sgl[][])
                                n770 = local write "img_CH2"(w3106) -> ()
                                n771 = local write "img_CH1"(w3098) -> ()
                                n772 = Quotient & Remainder(x=w3100, y=w3101) -> (floor(x/y)=→"photons/frame":i32)  [unwired: 1 out]
                                n773 = To Double Precision Float(number=w3104) -> (double precision float=w3103:dbl)
                                n774 = property on="img_CH1" class="IntGraph (strict)"("ZScale.Maximum"=w3103) -> ()  [unwired: 2 in, 2 out]
                                }
                                }
                                }
                                frame Enabled {
                                }
                                }
                                }
                                }
                                }
                                }
                                n775 = local read "save\ndata"() -> (w3089:bool)
                                n776 = case shown="True" w3089 {
                                frame False {
                                }
                                frame True {
                                n777 = local read "Current Average"() -> (w3108:sgl)
                                n778 = call "savetiffs.vi"("current average"=w3108) -> ()
                                }
                                }
                                }
                                frame #4 {
                                n779 = local read "save\ndata"() -> (w3109:bool)
                                n780 = case shown="True" w3109 {
                                frame False {
                                }
                                frame True {
                                n781 = local read "points recorded"() -> (w3111:i32)
                                n782 = call "timestamps.vi"("points recorded"=w3111, "command"="add") -> ()  [unwired: 2 in, 1 out]
                                }
                                }
                                }
                                frame #5 {
                                n783 = local read "Live"() -> (w3112:bool)
                                n784 = case shown="True" w3112 {
                                frame False {
                                }
                                frame True {
                                n785 = local read "downright"() -> (w3117:bool)
                                n786 = local read "downleft"() -> (w3119:bool)
                                n787 = local read "upright"() -> (w3115:bool)
                                n788 = local read "upleft"() -> (w3113:bool)
                                n789 = local read "down"() -> (w3118:bool)
                                n790 = local read "right"() -> (w3116:bool)
                                n791 = local read "left"() -> (w3120:bool)
                                n792 = local read "up"() -> (w3114:bool)
                                n793 = Compound Arithmetic op=OR(w3113, w3114, w3115, w3116, w3117, w3118, w3119, w3120) -> (w3121:bool)
                                n794 = case shown="True" w3121 {
                                frame False {
                                }
                                frame True {
                                n795 = stacked-sequence {
                                frame #0 {
                                n796 = local read "downright"() -> (w3123:bool)
                                n797 = local read "downleft"() -> (w3125:bool)
                                n798 = local read "BigSmall"() -> (w3122:bool)
                                n799 = local read "upright"() -> (w3127:bool)
                                n800 = local read "upleft"() -> (w3130:bool)
                                n801 = local read "down"() -> (w3126:bool)
                                n802 = local read "right"() -> (w3128:bool)
                                n803 = local read "left"() -> (w3124:bool)
                                n804 = local read "up"() -> (w3129:bool)
                                n805 = call "movestageparams.vi"("command"="get") -> ("Params out"=w3133:T22)  [unwired: 1 in]
                                n806 = Bundle By Name(cluster=w3133, "upleft"=w3130, "up"=w3129, "upright"=w3127, "right"=w3128, "downright"=w3123, "down"=w3126, "downleft"=w3125, "left"=w3124, "Bigsmall"=w3122) -> (w3134:T22)
                                n807 = call "movestageparams.vi"("Params in"=w3134, "command"="set") -> ()  [unwired: 1 out]
                                }
                                frame #1 {
                                n808 = call "movestage.vi"() -> ()  [unwired: 12 in]
                                }
                                frame #2 {
                                w3135 = FALSE ("OK Button")
                                w3136 = FALSE ("OK Button")
                                n809 = property on="down" class="Bool (strict)"("Value"=w3136) -> ()  [unwired: 2 in, 2 out]
                                n810 = property on="up" class="Bool (strict)"("Value"=w3136) -> ()  [unwired: 2 in, 2 out]
                                n811 = property on="right" class="Bool (strict)"("Value"=w3136) -> ()  [unwired: 2 in, 2 out]
                                n812 = property on="left" class="Bool (strict)"("Value"=w3136) -> ()  [unwired: 2 in, 2 out]
                                n813 = property on="upright" class="Bool (strict)"("Value"=w3135) -> ()  [unwired: 2 in, 2 out]
                                n814 = property on="downleft" class="Bool (strict)"("Value"=w3135) -> ()  [unwired: 2 in, 2 out]
                                n815 = property on="downright" class="Bool (strict)"("Value"=w3135) -> ()  [unwired: 2 in, 2 out]
                                n816 = property on="upleft" class="Bool (strict)"("Value"=w3135) -> ()  [unwired: 2 in, 2 out]
                                }
                                }
                                }
                                }
                                }
                                }
                                }
                                frame #6 {
                                n817 = local read "Live"() -> (w3139:bool)
                                n818 = case shown="True" w3139 {
                                tunnel: w3138 -> [_ w3146]
                                tunnel: w3137 -> [_ w3145]
                                frame False {
                                }
                                frame True {
                                n819 = local read "Laserpower \n(%)"() -> (w3141:dbl)
                                n820 = local read "lpow"() -> (w3140:dbl)
                                n821 = Not Equal?(x=w3140, y=w3146) -> (x != y?=w3142:bool)
                                n822 = Not Equal?(x=w3141, y=w3145) -> (x != y?=w3143:bool)
                                n823 = Or(x=w3143, y=w3142) -> (x .or. y?=w3144:bool)
                                n824 = case shown="True" w3144 {
                                tunnel: w3143 -> [_ w3150]
                                tunnel: w3142 -> [_ w3149]
                                tunnel: w3141 -> [_ w3148]
                                tunnel: w3140 -> [_ w3147]
                                frame False {
                                }
                                frame True {
                                n825 = case shown="True" w3150 {
                                tunnel: w3148 -> [_ w3153]
